vi "SymmetricFunc.FitFunc.vi"(3 "output control":T1, 4 "data":variant, 5 "X":dbl[](array[numeric]), 6 "Coefficients":dbl[](array[numeric])) -> (0 "error out":errorcluster, 1 "f'(X,a)":dbl[][](array[numeric]), 2 "f(X,a)":dbl[](array[numeric]))   [LabVIEW 2020, in "XYcenter.lvlib"]
uses:
  XYcenter.lvlib
  <vilib>/gmath/NumericalOptimization/LM_output select.ctl
  <vilib>/gmath/NI_Gmath.lvlib
panel:
  out "sum":dbl
  out "Waveform Chart":dbl(graph)
  out "data and fit 2":cluster{dbl[], dbl[]}(graph)
  out "data and fit":cluster{dbl[], "Best Polynomial Fit":dbl[]}[](graph)
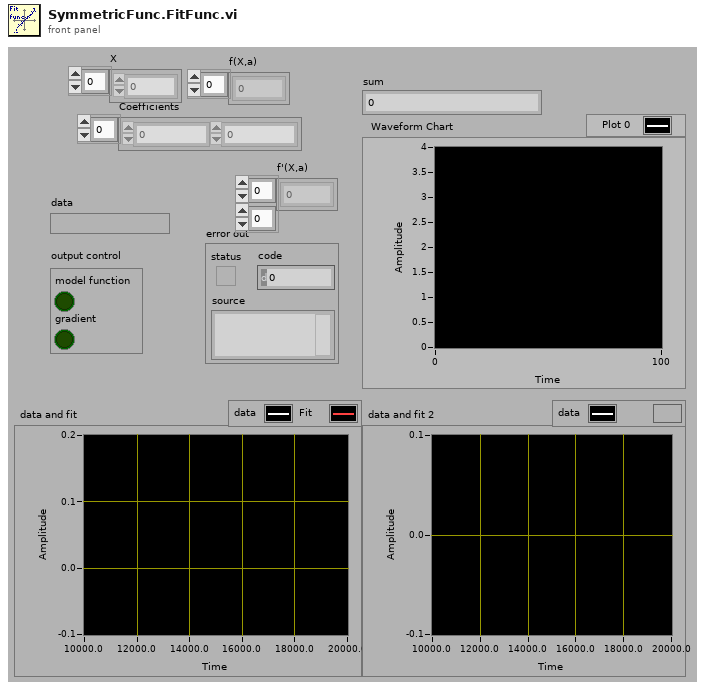
[diagram p1: front panel]
types:
  T1 = typedef "NI_Gmath.lvlib/LM_output select.ctl" = cluster{"model function":bool, "gradient":bool}
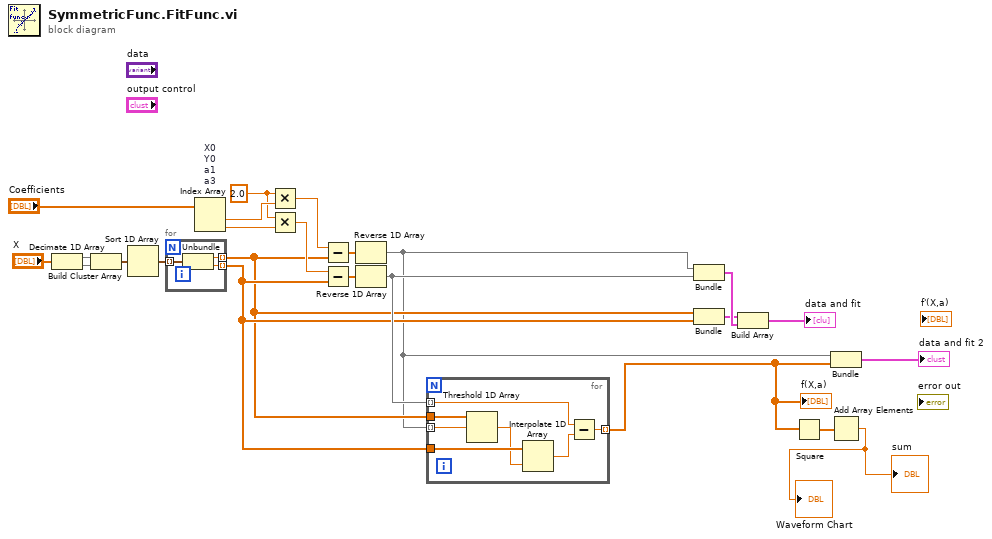
[diagram p0: block diagram]
diagram:
  w21 = 2.0 ("y")
  n1 = Decimate 1D Array("X") -> (w14:dbl[], w13:dbl[])
  n2 = Build Cluster Array(w14, w13) -> (w12:cluster{"x":dbl, "x":dbl}[])
  n3 = Sort 1D Array(array=w12) -> (sorted array=w11:cluster{"x":dbl, "x":dbl}[])
  n4 = for {
    tunnel: w11 -> [w27] mode=indexing
    tunnel: [w26] -> w2 mode=indexing
    tunnel: [w25] -> w3 mode=indexing
    n5 = Unbundle(w27) -> ("x"=w26:dbl, "x"=w25:dbl)
  }
  n6 = Index Array "X0\nY0\na1\na3"(array="Coefficients") -> (element #1=w22:dbl, element #2=w20:dbl)  [unwired: 2 in]
  n7 = Multiply(x=w21, y=w22) -> (x*y=w19:dbl)
  n8 = Multiply(x=w21, y=w20) -> (x*y=w18:dbl)
  n9 = Subtract(x=w19, y=w2) -> (x-y=w10:dbl[])
  n10 = Subtract(x=w18, y=w3) -> (x-y=w9:dbl[])
  n11 = Reverse 1D Array(array=w10) -> (reversed array=w1:dbl[])
  n12 = Reverse 1D Array(array=w9) -> (reversed array=w4:dbl[])
  n13 = for {
    tunnel: w2 -> [w34]
    tunnel: w3 -> [w33]
    tunnel: w1 -> [w32] mode=indexing
    tunnel: w4 -> [w31] mode=indexing
    tunnel: [w29] -> w7 mode=indexing
    n14 = Threshold 1D Array(2:w32, 3:w34) -> (0:w28:dbl)  [unwired: 1 in]
    n15 = Interpolate 1D Array(1:w28, 2:w33) -> (0:w30:dbl)
    n16 = Subtract(x=w31, y=w30) -> (x-y=w29:dbl)
  }
  "f(X,a)" <- w7
  n17 = Bundle(w1, w4) -> (w17:cluster{dbl[], dbl[]})  [unwired: 1 in]
  n18 = Bundle(w2, w3) -> (w16:cluster{dbl[], dbl[]})  [unwired: 1 in]
  n19 = Build Array(w16, w17) -> (→"data and fit":cluster{dbl[], dbl[]}[])
  n20 = Square(x=w7) -> (x^2=w6:dbl[])
  n21 = Bundle(w1, w7) -> (→"data and fit 2":cluster{dbl[], dbl[]})  [unwired: 1 in]
  n22 = Add Array Elements(numeric array=w6) -> (sum=→"Waveform Chart" →"sum":dbl)
